vi "rqcAlice SPI PM Level test (Host).vi"() -> ()   [LabVIEW 2018]
uses:
  Shared/Shared FPGA Lib/Shared Logic/Custom Controls/rqc Random Generator.parameters.ctl
  Shared/Shared FPGA Lib/Shared Logic/Custom Controls/rqc Random Generator.value type.ctl
  <vilib>/FPGAPlugInAG/PCIe-7820R/niLvFpga_Open_PCIe-7820R.vi
  <vilib>/rvi/interface/common/dynamic/niFpgaDynamicAddResources.vi
  <vilib>/Utility/error.llb/Error Cluster From Error Code.vi
  <vilib>/rvi/errors/niLvFpgaAdjustHostInterfaceError.vi
  <vilib>/FPGAPlugInAG/Dynamic/niLvFpga_Close_Dynamic.vi
  <vilib>/rvi/interface/nirviOpenFPGA/nirviOpenFPGA.xnode
  FPGA Bitfiles/rqcAlice SPI PM Level test 1.0.0.lvbitx
  <vilib>/rvi/interface/nirviReadWriteControl/nirviReadWriteControl.xnode
  <vilib>/rvi/interface/nirviCloseFPGA/nirviCloseFPGA.xnode
  NiFpgaLv.dll
  <vilib>/rvi/interface/Simulation/niFpgaSimulationCallBeginRW.vi
panel:
  out "Array":u32[](array[numeric]) format="%024b"
  out "error out":errorcluster
  in  "level":u8
  in  "Send to DAC":bool
  in  "Update Values":bool
  in  "RndGen.parameters":T1={"value type"=enum."constant", "constant"=0, "num of levels"=0, "levels values"=[0, 0, 0, 0]}
  in  "stop":bool
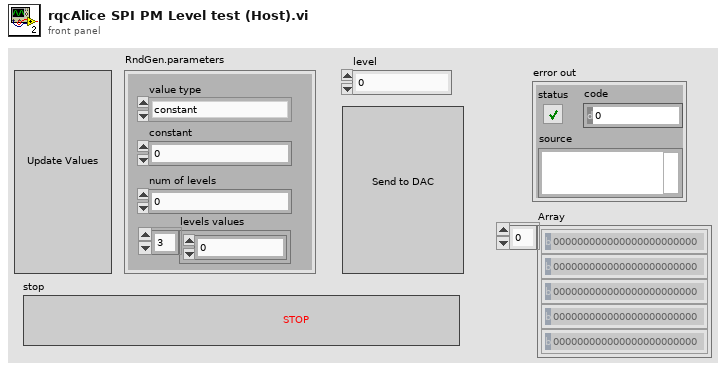
[diagram p1: front panel]
types:
  T1 = typedef "rqc Random Generator.parameters.ctl" = cluster{"value type":T2, "constant":u16, "num of levels":u16, "levels values":u16[]}
  T2 = typedef "rqc Random Generator.value type.ctl" = enum16{"random value", "constant"}
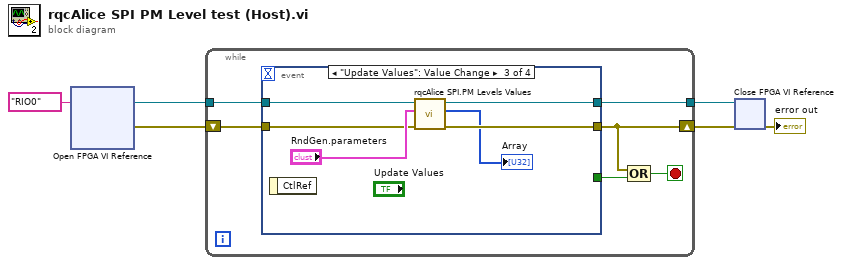
[diagram p0: block diagram]
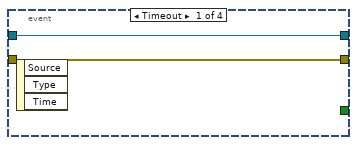
[diagram p2: hidden frame]
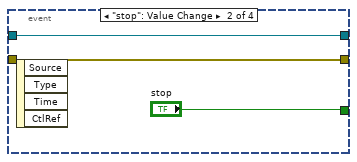
[diagram p3: hidden frame]
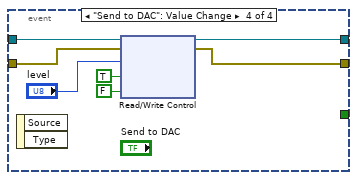
[diagram p4: hidden frame]
diagram:
  n1 = xnode "Open FPGA VI Reference"("resource name"=tag "RIO0") -> ("FPGA VI Reference Out"=w5:refnum<k20>, "error out"=w4:errorcluster)  [unwired: 1 in]
  n2 = while {
    tunnel: w5 -> [w12]
    tunnel: [w11] -> w3
    shift-right: [w7] -> w2
    shift-left: w4 -> [w10]
    stop <- w8 stop-if-true
    n3 = event shown="[2] \"Update Values\": Value Change" {
      selector: _ -> [_ _ _ _]
      dyn-events: _ -> [_ _ _ _]
      timeout: _ -> [_ _ _ _]
      tunnel: w12 -> [w14 w15 w22 w30]
      tunnel: [w14 w15 w21 w24] -> w11
      tunnel: [w13 w16 w19 w25] -> w7
      tunnel: w10 -> [w13 w16 w20 w26]
      tunnel: [_ "stop" _ _] -> w9
      event Timeout {
        n4 = event-data() -> ()  [unwired: 1 in, 3 out]
      }
      event "stop": Value Change {
        n5 = event-data() -> ()  [unwired: 1 in, 4 out]
      }
      event "Update Values": Value Change {
        n6 = event-data() -> ()  [unwired: 1 in, 1 out]
        n7 = call "rqcAlice SPI.PM Levels Values.vi"("error in"=w20, "RndGen.parameters"="RndGen.parameters", "Alice FPGA Reference In"=w22) -> ("error out"=w19:errorcluster, "data writen"=→"Array":u32[], "Alice FPGA Reference Out"=w21:refnum<k20>)  [unwired: 6 in]
      }
      event "Send to DAC": Value Change {
        n8 = event-data() -> ()  [unwired: 1 in, 2 out]
        n9 = xnode "Read/Write Control"("FPGA VI Reference In"=w30, "error in"=w26, "level"="level", "send clock"=TRUE, "send clock"=FALSE) -> ("FPGA VI Reference Out"=w24:refnum<k20>, "error out"=w25:errorcluster)
      }
    }
    n10 = Compound Arithmetic op=OR(w7, w9) -> (w8:bool)
  }
  n11 = xnode "Close FPGA VI Reference"("FPGA VI Reference In"=w3, "error in"=w2) -> ("error out"=→"error out":errorcluster)
